vi "Append to Array - Known Type.vi"(5 "JSON Compatible Type":T1=enum."Unknown", 6 "Add Parameter as JSON Tree?":bool, 7 "JSON Type":T2=enum."Unknown", 8 "error in (no error)":errorcluster, 10 "Value":variant, 11 "JSON Tree in (JSON Array)":variant) -> (0 "error out":errorcluster, 3 "JSON Tree out (JSON Array)":variant)   [LabVIEW 2013, in "i3-json.lvlib"]
doc: "Appends a known value to the given array"
uses:
  i3-json.lvlib
  JSON Types/JSON Type.ctl
  JSON Types/JSON Compatible Type.ctl
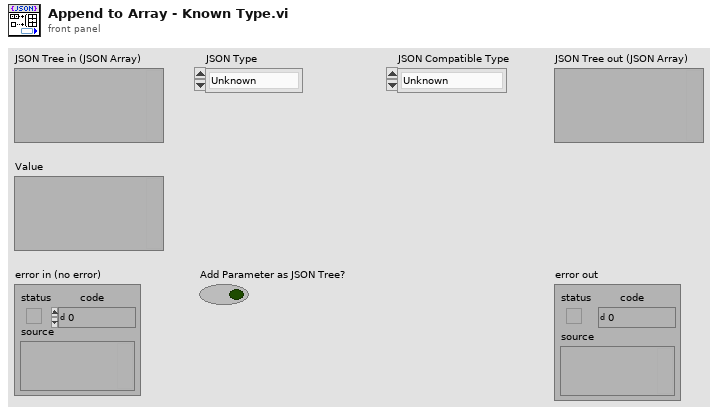
[diagram p1: front panel]
types:
  T1 = typedef "i3-json.lvlib/JSON Compatible Type.ctl" = enum16{"1D Double Array", "1D String Array", "1D Boolean Array", "Unknown"}
  T2 = typedef "i3-json.lvlib/JSON Type.ctl" = enum8{"JSON Compatible", "JSON Array", "JSON Object", "JSON Null", "Double", "String", "Boolean", "Unknown"}
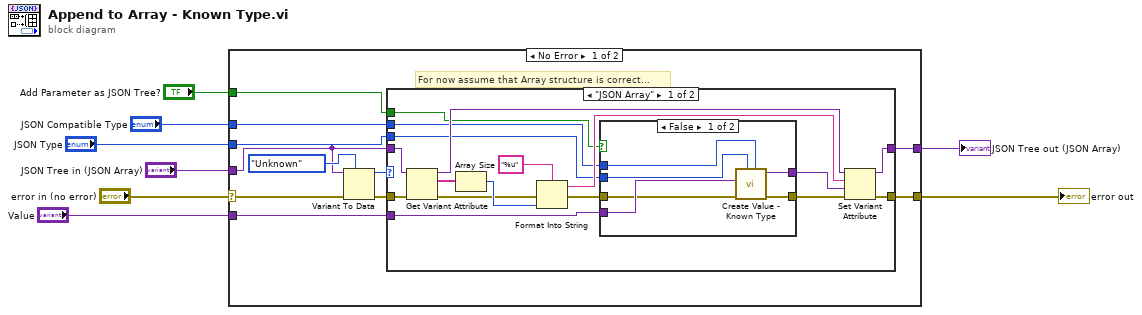
[diagram p0: block diagram]
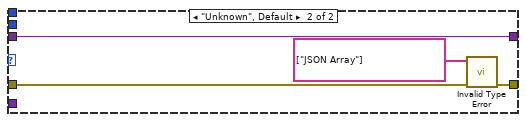
[diagram p3: hidden frame]
diagram:
  n1 = case shown="No Error" "error in (no error)" {
    selector: "error in (no error)" -> [w17 w50]
    tunnel: [w15 w50] -> w7
    tunnel: [w14 w49] -> w6
    tunnel: "JSON Tree in (JSON Array)" -> [w13 w49]
    tunnel: "Add Parameter as JSON Tree?" -> [w12 _]
    tunnel: "Value" -> [w11 _]
    tunnel: "JSON Type" -> [w10 _]
    tunnel: "JSON Compatible Type" -> [w9 _]
    frame No Error {
      # "For now assume that Array structure is correct..."
      n2 = Variant To Data(error in=w17, type=JSON_Type."Unknown" ("JSON Type"), Variant=w13) -> (data=w18:T2, error out=w16:errorcluster)
      n3 = case shown="\"JSON Array\"" w18 {
        tunnel: w13 -> [w35 w48]
        tunnel: w16 -> [w34 w46]
        tunnel: [w25 w48] -> w14
        tunnel: [w24 w45] -> w15
        tunnel: w12 -> [w23 _]
        tunnel: w11 -> [w22 _]
        tunnel: w10 -> [w21 _]
        tunnel: w9 -> [w20 _]
        frame "JSON Array" {
          n4 = Get Variant Attribute(Variant=w35, error in=w34) -> (duplicate Variant=w33:variant, names=w36:string[], error out=w31:errorcluster)  [unwired: 2 in, 1 out]
          n5 = Array Size(array=w36) -> (size(s)=w32:i32)
          n6 = Format Into String(format string="%u", error in=w31, w32) -> (resulting string=w29:string, error out=w28:errorcluster)  [unwired: 1 in]
          n7 = case shown="False" w23 {
            tunnel: w22 -> [w42 w44]
            tunnel: w28 -> [w41 w43]
            tunnel: [w40 w43] -> w27
            tunnel: [w39 w44] -> w26
            tunnel: w21 -> [w38 _]
            tunnel: w20 -> [w37 _]
            frame False {
              n8 = call "Create Value - Known Type.vi"("JSON Compatible Type"=w37, "JSON Type"=w38, "error in (no error)"=w41, "Value"=w42) -> ("error out"=w40:errorcluster, "JSON Tree"=w39:variant)  [unwired: 6 in]
            }
            frame True {
              # "ASSUMES VALID\nJSON TREE - maybe\nshould run-time check?"
            }
          }
          n9 = Set Variant Attribute(Variant=w33, name=w29, value=w26, error in=w27) -> (Variant out=w25:variant, error out=w24:errorcluster)  [unwired: 1 out]
        }
        frame "Unknown", Default {
          n10 = call "Invalid Type Error.vi"("error in (no error)"=w46, "Valid Types"=string[] ["JSON Array"]) -> ("error out"=w45:errorcluster)  [unwired: 9 in]
        }
      }
    }
    frame Error {
    }
  }
  "error out" <- w7
  "JSON Tree out (JSON Array)" <- w6
